vi "PFI-28000-System_Parse Config String.vi"(0 "Line":string, 11 "error in (no error)":errorcluster) -> (4 "Frame":i32, 6 "Slot":i32, 8 "Model":string, 10 "SN":string, 14 "Channels":i32[](array[numeric]), 15 "error out":errorcluster)   [LabVIEW 2017, in "PFI-28000-System.lvclass"]
uses:
  PFI-28000-System.lvclass
  <vilib>/regexp/Match Regular Expression.xnode
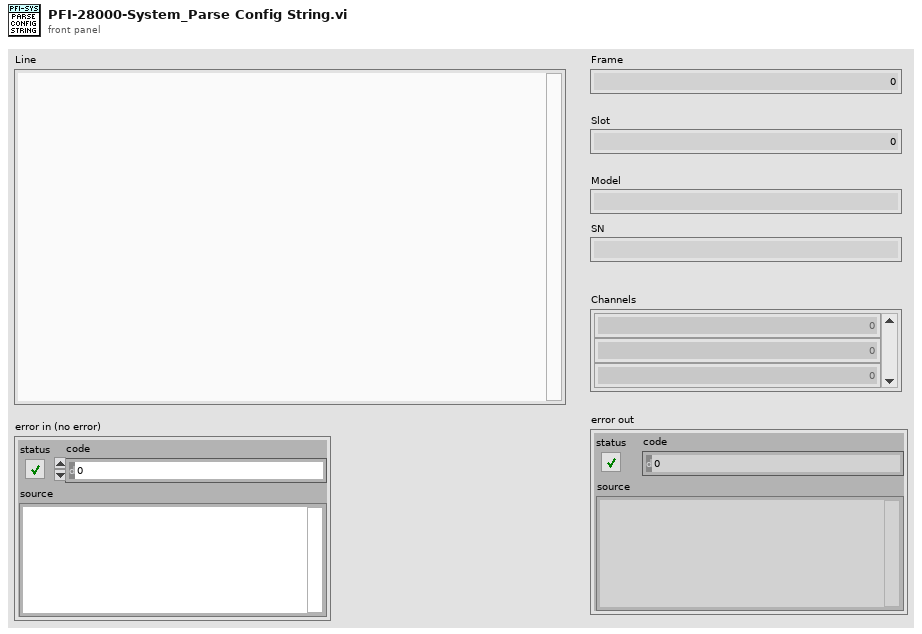
[diagram p1: front panel]
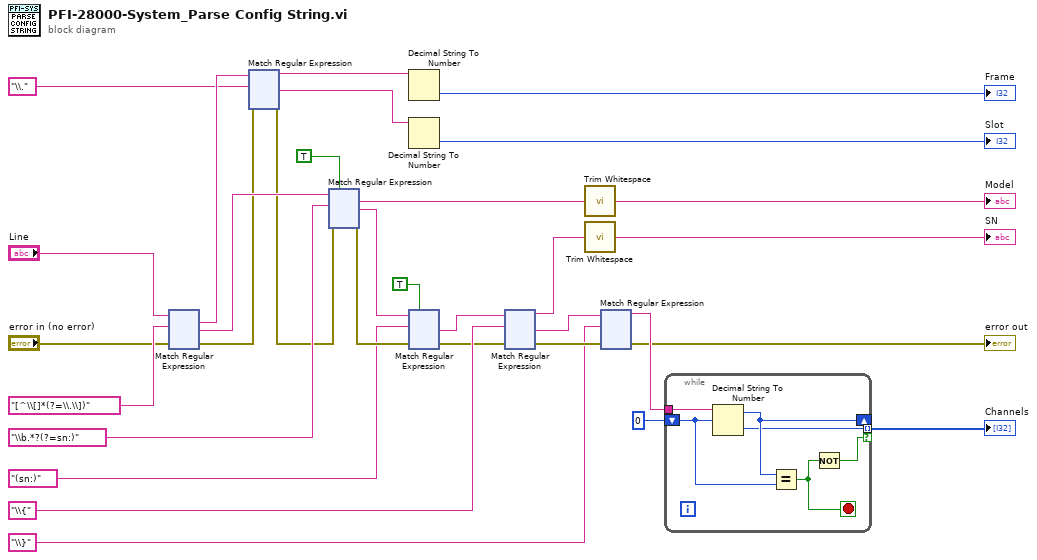
[diagram p0: block diagram]
diagram:
  n1 = xnode "Match Regular Expression"("input string"="Line", "regular expression"="[^\\[]*(?=\\.\\])" ("empty string"), "error in"="error in (no error)") -> ("whole match"=w30:string, "after match"=w25:string, "error out"=w16:errorcluster)  [unwired: 3 in, 2 out]
  n2 = xnode "Match Regular Expression"("input string"=w30, "regular expression"="\\." ("empty string"), "error in"=w16) -> ("before match"=w28:string, "after match"=w23:string, "error out"=w15:errorcluster)  [unwired: 3 in, 2 out]
  n3 = xnode "Match Regular Expression"("input string"=w25, "regular expression"="\\b.*?(?=sn:)" ("empty string"), "error in"=w15, "ignore case? (F)"=TRUE) -> ("whole match"=w19:string, "after match"=w21:string, "error out"=w17:errorcluster)  [unwired: 2 in, 2 out]
  n4 = Decimal String To Number(string=w28) -> (number=→"Frame":i32)  [unwired: 2 in, 1 out]
  n5 = Decimal String To Number(string=w23) -> (number=→"Slot":i32)  [unwired: 2 in, 1 out]
  n6 = xnode "Match Regular Expression"("input string"=w21, "regular expression"="(sn:)" ("empty string"), "error in"=w17, "ignore case? (F)"=TRUE) -> ("after match"=w13:string, "error out"=w9:errorcluster)  [unwired: 2 in, 3 out]
  n7 = xnode "Match Regular Expression"("input string"=w13, "regular expression"="\\{" ("empty string"), "error in"=w9) -> ("before match"=w11:string, "after match"=w7:string, "error out"=w8:errorcluster)  [unwired: 3 in, 2 out]
  n8 = call <vilib>:"Trim Whitespace.vi"("string"=w19) -> ("trimmed string"=→"Model":string)  [unwired: 1 in]
  n9 = call <vilib>:"Trim Whitespace.vi"("string"=w11) -> ("trimmed string"=→"SN":string)  [unwired: 1 in]
  n10 = xnode "Match Regular Expression"("input string"=w7, "regular expression"="\\}" ("empty string"), "error in"=w8) -> ("before match"=w4:string, "error out"=→"error out":errorcluster)  [unwired: 3 in, 3 out]
  n11 = while {
    shift-right: [w37] -> _
    shift-left: 0 ("offset (0)") -> [w33]
    tunnel: w4 -> [w38]
    tunnel: [w36] -> w3 mode=indexing if=w35
    stop <- w34 stop-if-true
    n12 = Decimal String To Number(string=w38, offset=w33) -> (offset past number=w37:i32, number=w36:i32)  [unwired: 1 in]
    n13 = Equal?(x=w37, y=w33) -> (x = y?=w34:bool)
    n14 = Not(x=w34) -> (.not. x?=w35:bool)
  }
  "Channels" <- w3
